vi "remove.vi"() -> ()   [LabVIEW 2018]
uses:
  TcpServer.lvclass
panel:
  out "Array":string[](array[string])
  in  "evtDetails":string="\"InPoistion\" : True\n\n\"Tolerance\" : 0.1"
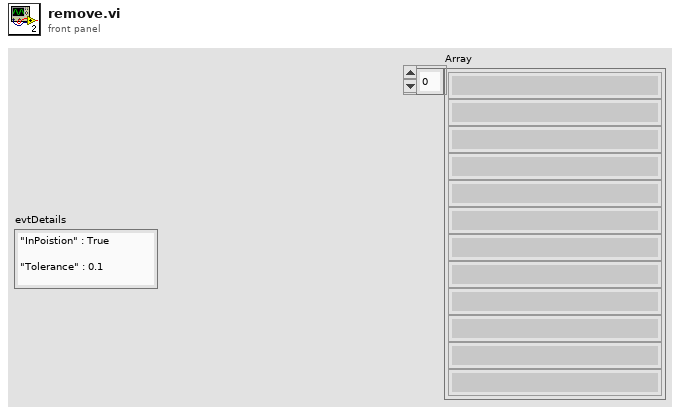
[diagram p1: front panel]
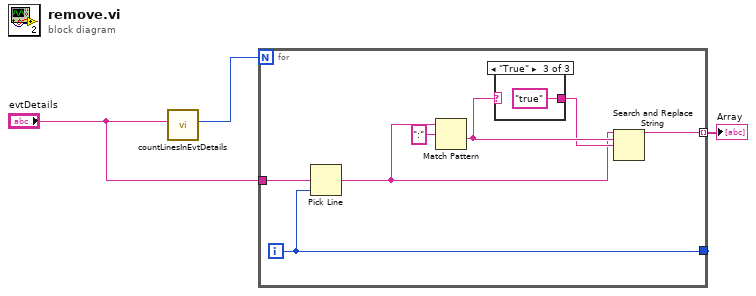
[diagram p0: block diagram]
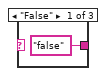
[diagram p2: hidden frame]
diagram:
  n1 = call "countLinesInEvtDetails.vi"("evtDetails"="evtDetails") -> ("numberOfLines"=w3:i32)  [unwired: 9 in, 1 out]
  n2 = for {
    N: w3 -> [_]
    tunnel: "evtDetails" -> [w10]
    tunnel: [w9] -> _
    tunnel: [w4] -> w1 mode=indexing
    i -> [w9]
    n3 = Pick Line(multi-line string=w10, line index=w9) -> (output string=w5:string)  [unwired: 1 in]
    n4 = Match Pattern(string=w5, regular expression=":") -> (after substring=w7:string)  [unwired: 1 in, 3 out]
    n5 = case shown="\"True\"" w7 {
      selector: w7 -> [_ w12 _]
      tunnel: ["false" ("regular expression") w12 "true" ("regular expression")] -> w6
      frame "False" {
      }
      frame Default {
      }
      frame "True" {
      }
    }
    n6 = Search and Replace String(input string=w5, search string=w7, replace string=w6) -> (result string=w4:string)  [unwired: 5 in, 3 out]
  }
  "Array" <- w1
